vi "Install Dependencies.vi"(7 "Stored Install Data":path, 10 "Variant":variant) -> (0 "Error Out":errorcluster)   [LabVIEW 2011, in "LVH-Toolbox.lvlib" / "Installer Tools.lvlib"]
uses:
  Installer Tools.lvlib
  Private/Type Defs/Deps State.ctl
  <vilib>/Utility/file.llb/Read From Spreadsheet File (string).vi
  Private/Dependency Test VI Template.vi
  Common/LVH-Common.lvlib
panel:
  out "Tab Control":T1(tab)
  out "Package Name":string
  in  "Listbox":i32(listbox)
  in  "Info Cancel Button":bool
  in  "Info Next Button":bool
  out "Status":string
  out "Download Progress":u8(slide) scale=0.0..100.0
  in  "Multicolumn Listbox":i32(listbox)
  in  "Install Next":bool
  in  "Install Cancel":bool
  in  "Summary Finish":bool
  # "Testing Dependencies . . ."
  # "Select dependencies you want to install."
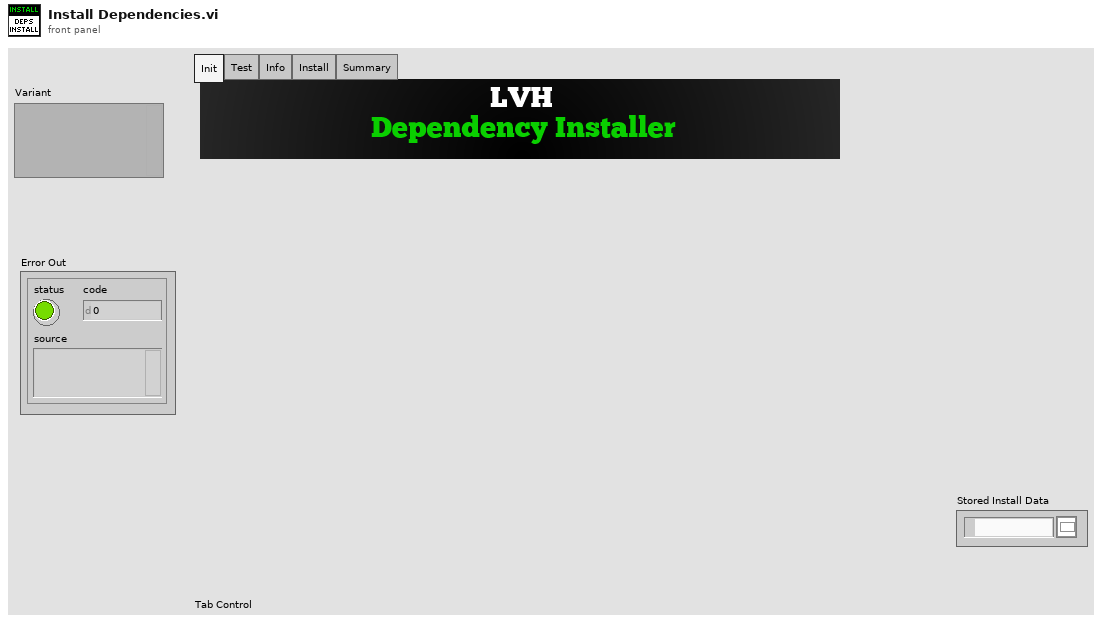
[diagram p1: front panel]
types:
  T1 = enum32{"Init", "Test", "Info", "Install", "Summary"}
  T2 = typedef "LVH-Toolbox.lvlib/Installer Tools.lvlib/Deps State.ctl" = enum16{"Init", "Test", "Info", "Install", "Summary"}
  T3 = typedef "LVH-Toolbox.lvlib/Installer Tools.lvlib/Dependency Config.ctl" = cluster{"Dependencies":T4[], "Files Installed":path[], "Dependency Config":path, "Installer Helper":path, "Dep Index":i32, "Download":T5}
  T4 = typedef "LVH-Toolbox.lvlib/Installer Tools.lvlib/Dependecy.ctl" = cluster{"Name":string, "Version":string, "Test VI Path":path, "Source URL":string, "Dep Met?":bool, "Install?":bool, "Installer Args":string}
  T5 = typedef "LVH-Toolbox.lvlib/LVH-Common.lvlib/Download Task.ctl" = cluster{"URL":string, "Local Path":path, "Download Worker":refnum<vi>, "Total Size (Bytes)":u64, "Prev Downloaded Size":u64, "Prev Download Time Stamp":timestamp}
  T6 = enum16{"Init", "Start DL", "Downloading", "DL Complete", "Done"}
  T7 = typedef "LVPoint32TypeDef.ctl" = cluster{"Horizontal":i32, "Vertical":i32}
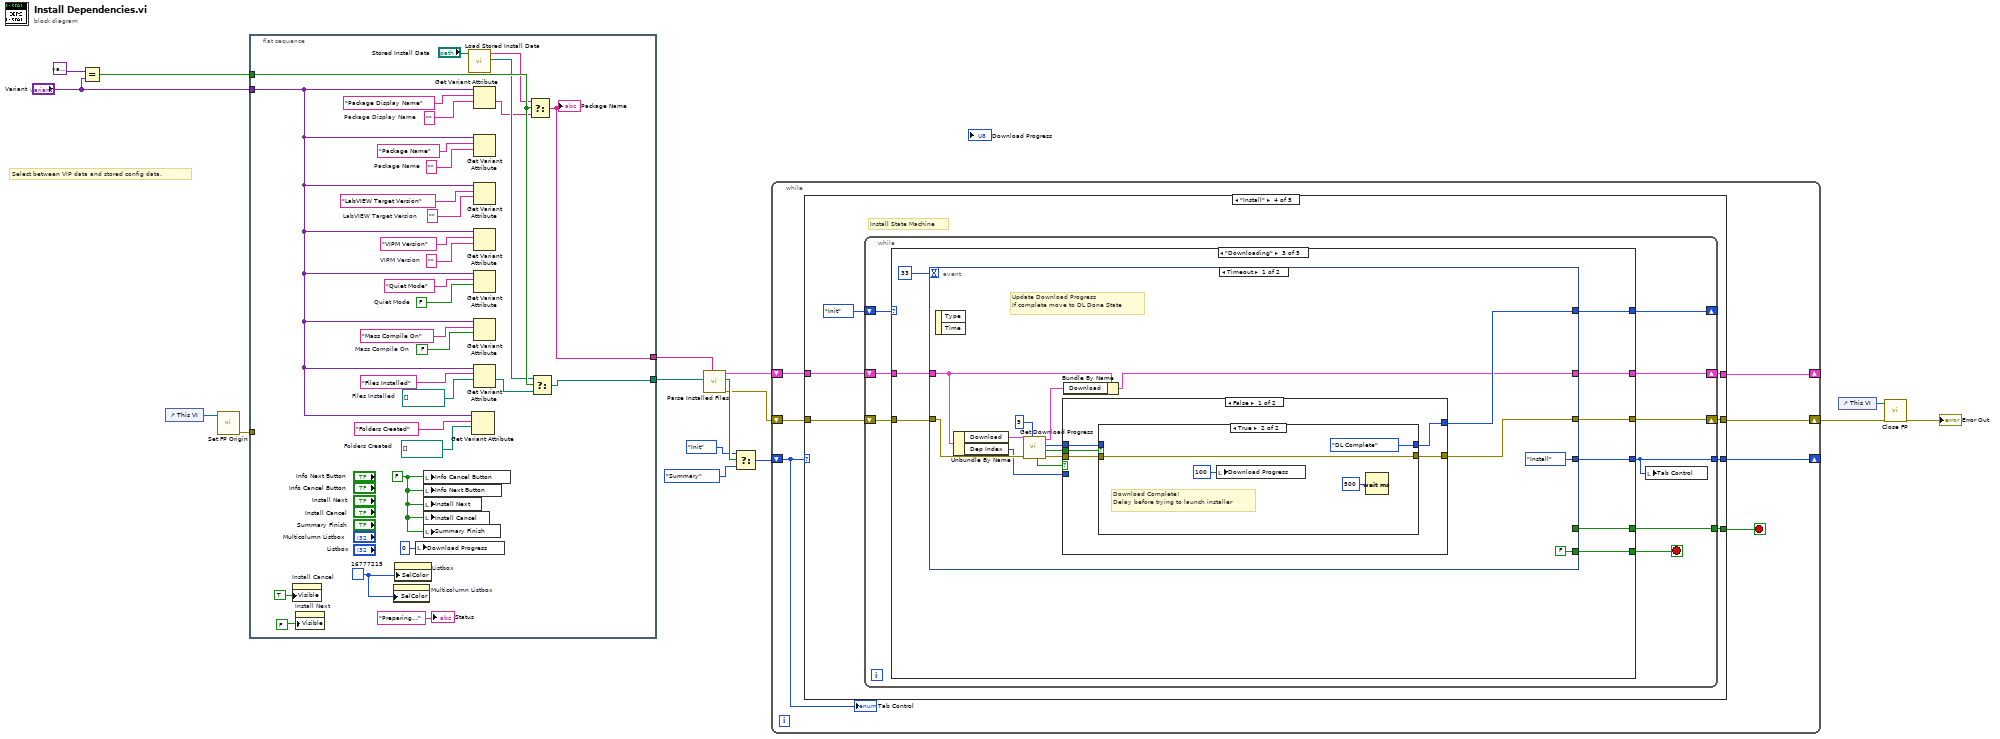
[diagram p0: block diagram]
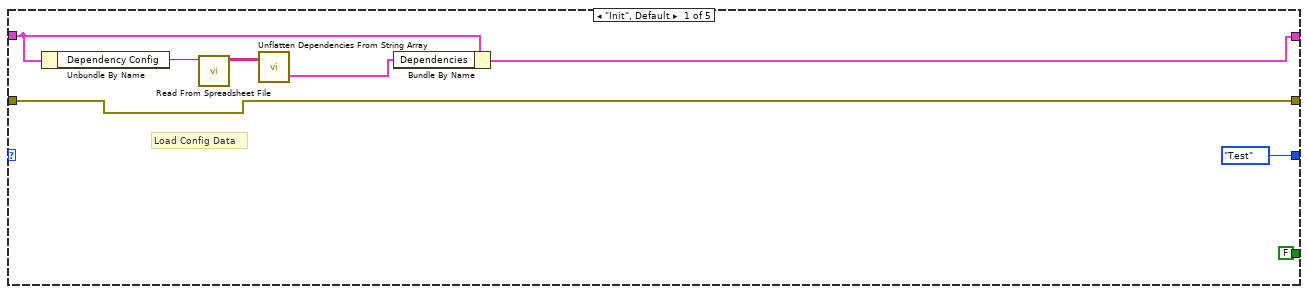
[diagram p2: hidden frame]
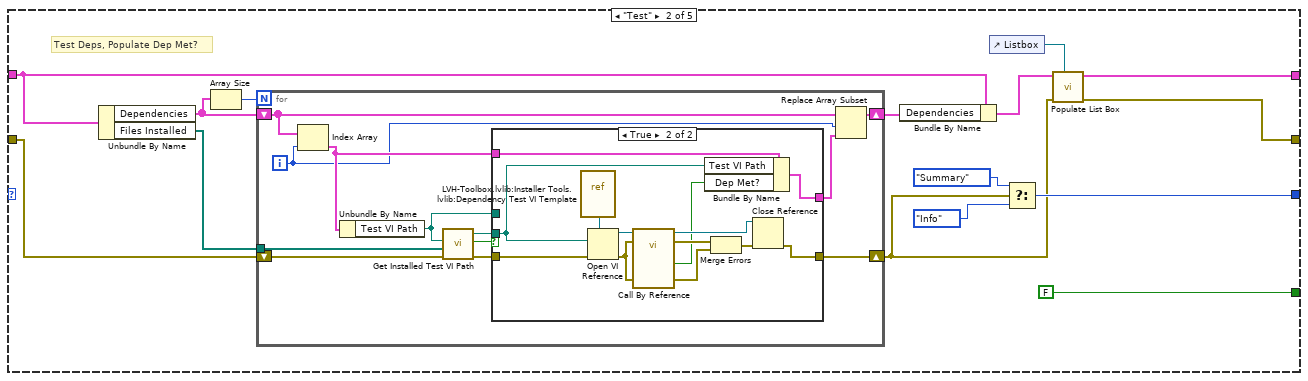
[diagram p3: hidden frame]
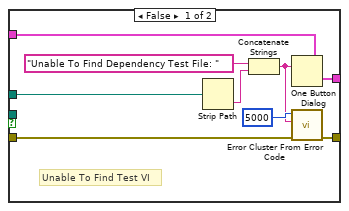
[diagram p4: hidden frame]
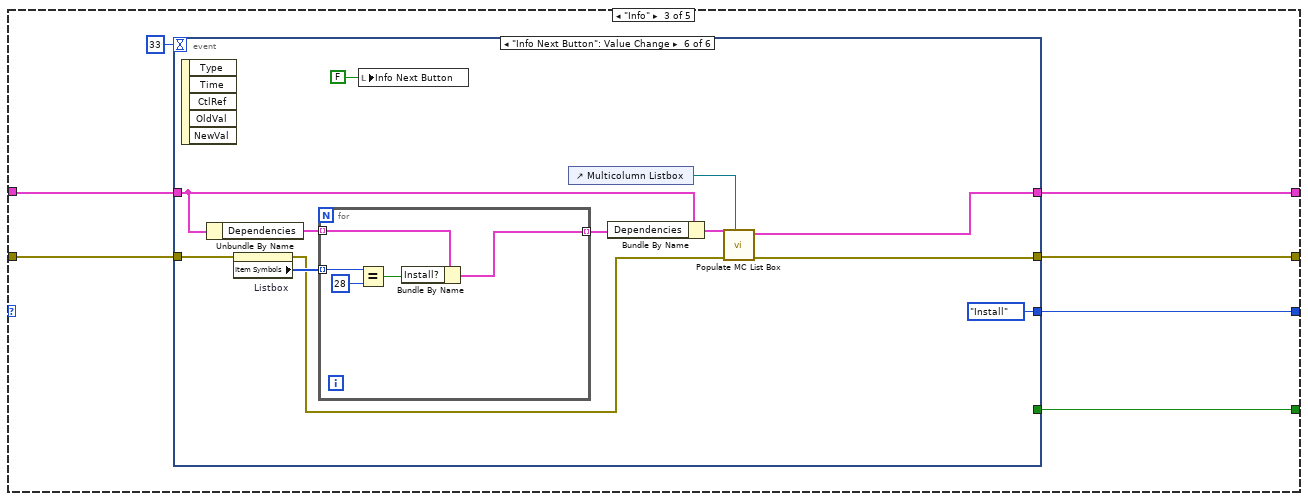
[diagram p5: hidden frame]
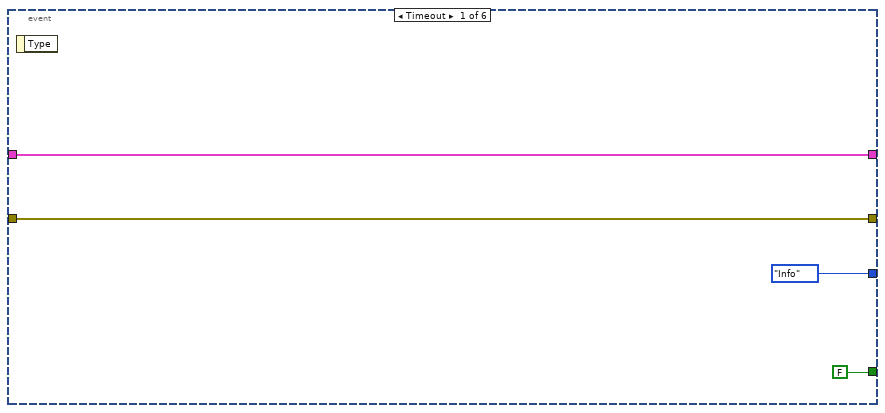
[diagram p6: hidden frame]
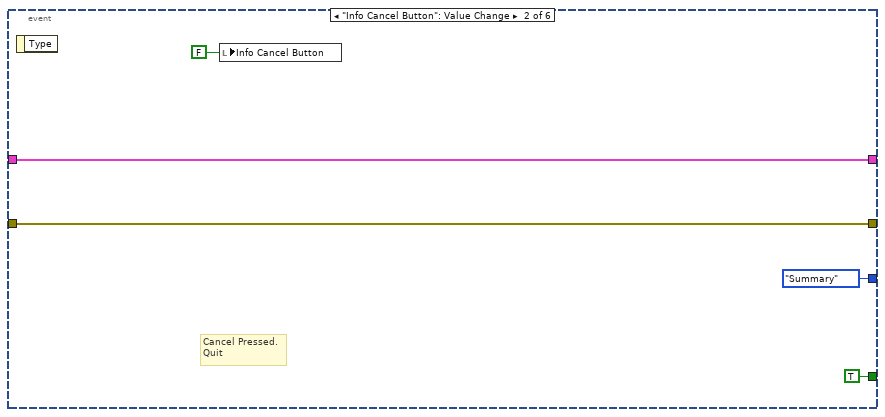
[diagram p7: hidden frame]
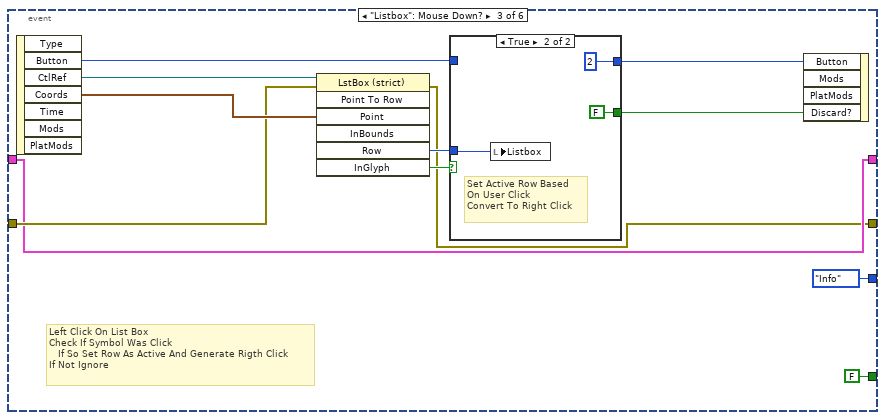
[diagram p8: hidden frame]
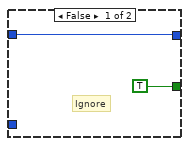
[diagram p9: hidden frame]
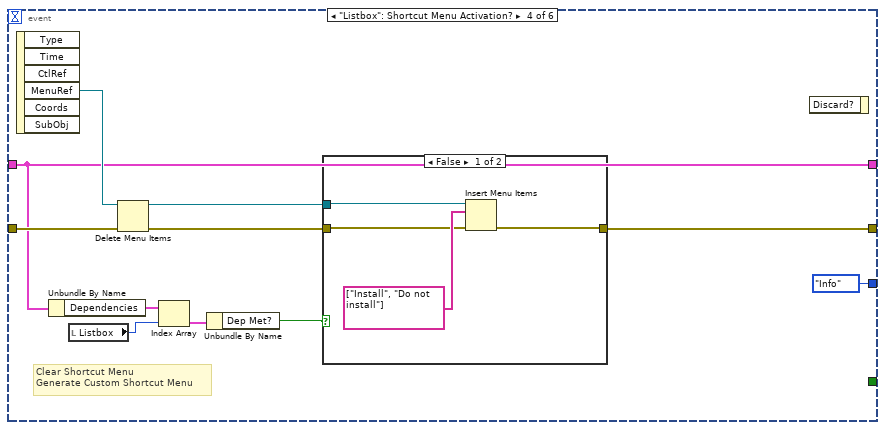
[diagram p10: hidden frame]
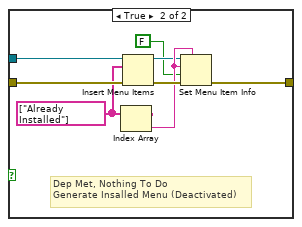
[diagram p11: hidden frame]
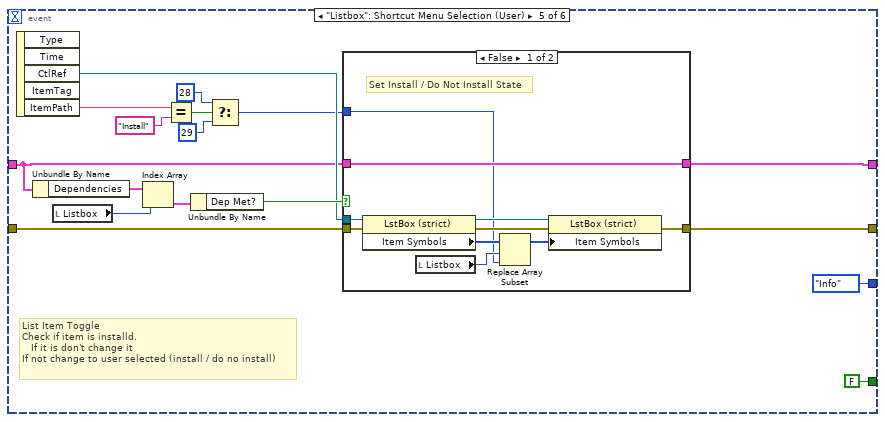
[diagram p12: hidden frame]
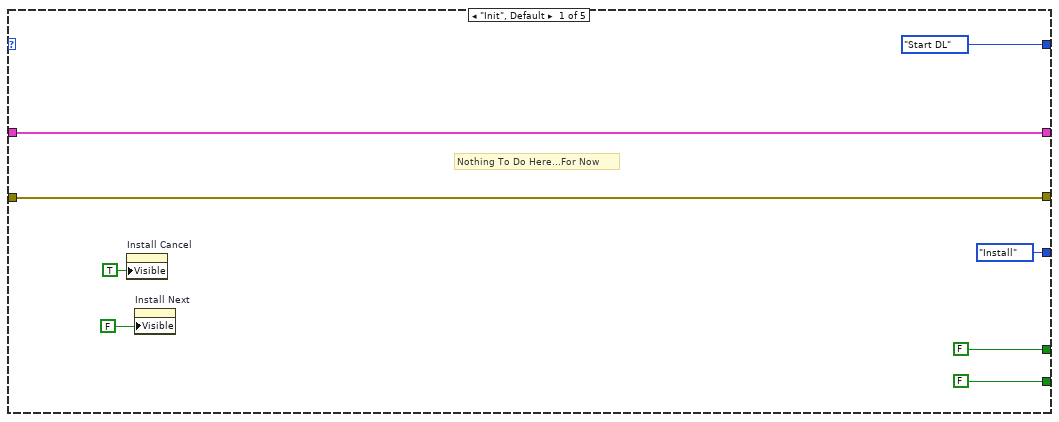
[diagram p14: hidden frame]
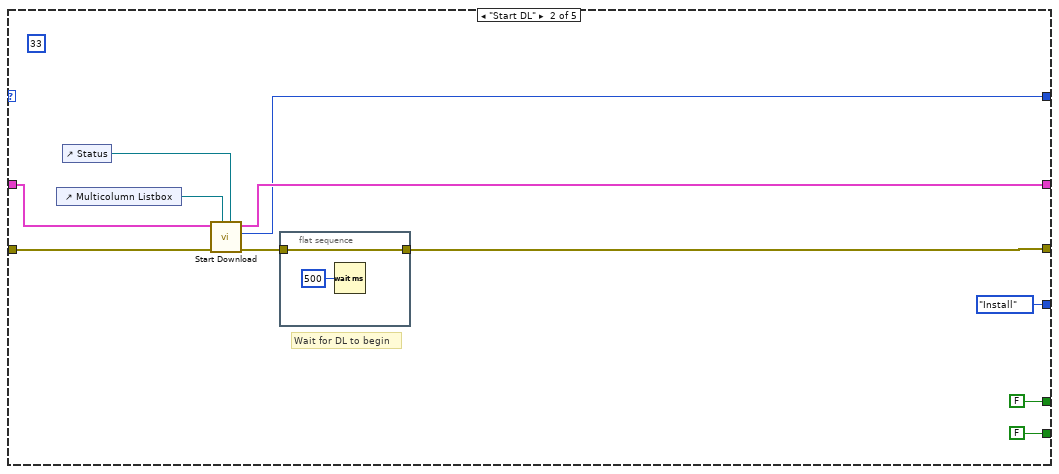
[diagram p15: hidden frame]
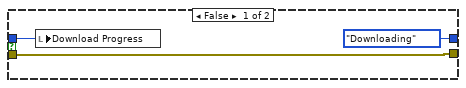
[diagram p16: hidden frame]
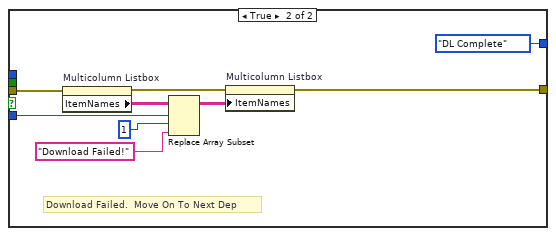
[diagram p17: hidden frame]
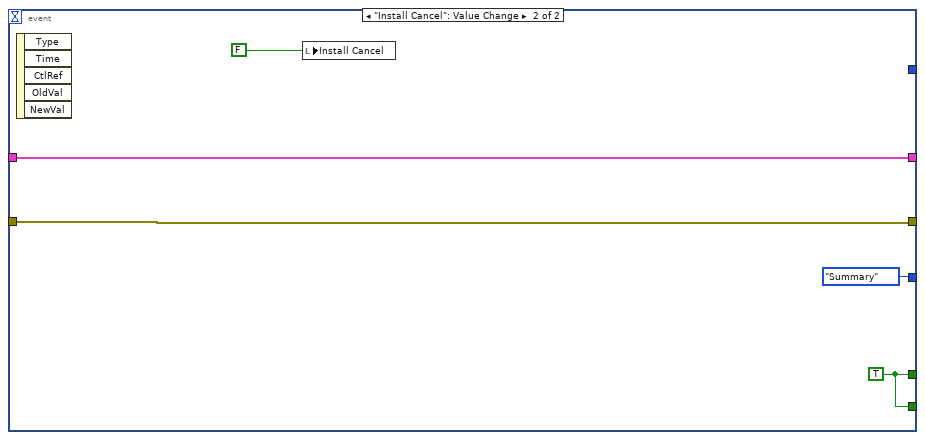
[diagram p18: hidden frame]
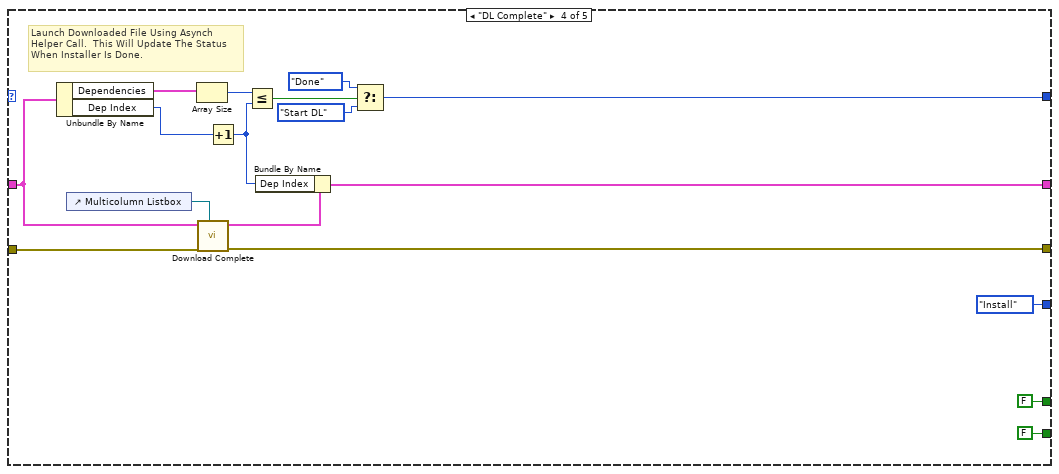
[diagram p19: hidden frame]
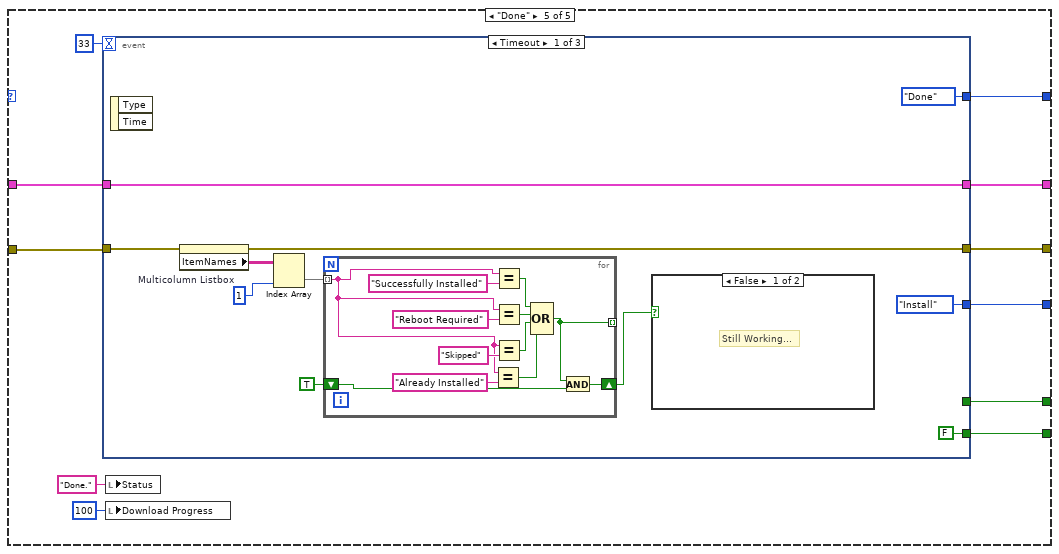
[diagram p20: hidden frame]
diagram:
  # "Select between VIP data and stored config data."
  n1 = Equal?(x=variant ("Variant"), y="Variant") -> (x = y?=w2:bool)
  n2 = control-ref of="This VI"() -> (w10:refnum<vi>)
  n3 = call "Set FP Origin.vi"("VI Ref"=w10) -> ("Error Out"=w11:errorcluster)  [unwired: 10 in]
  n4 = flat-sequence {
    tunnel: w11 -> [_]
    tunnel: "Variant" -> [w25]
    tunnel: [w21] -> w4
    tunnel: w2 -> [w24]
    tunnel: [w22] -> w1
    frame #0 {
      w31 = u32 16777215
      w29 = FALSE ("Cancel Button")
      w32 = path[] []  # Folders Created
      w33 = path[] []  # Files Installed
      w36 = FALSE  # Mass Compile On
      w37 = ""  # Package Display Name
      w38 = FALSE  # Quiet Mode
      w41 = ""  # VIPM Version
      w43 = ""  # LabVIEW Target Version
      w45 = ""  # Package Name
      n5 = property on="Install Cancel" class="Bool (strict)"("Visible"=TRUE) -> ()  [unwired: 2 in, 2 out]
      n6 = property on="Install Next" class="Bool (strict)"("Visible"=FALSE) -> ()  [unwired: 2 in, 2 out]
      n7 = property on="Multicolumn Listbox" class="MCListbox (strict)"("SelColor"=w31) -> ()  [unwired: 2 in, 2 out]
      n8 = property on="Listbox" class="LstBox (strict)"("SelColor"=w31) -> ()  [unwired: 2 in, 2 out]
      n9 = local write "Download Progress"(u8 0 ("Download Progress")) -> ()
      n10 = local write "Info Cancel Button"(w29) -> ()
      n11 = local write "Info Next Button"(w29) -> ()
      n12 = local write "Install Next"(w29) -> ()
      n13 = local write "Install Cancel"(w29) -> ()
      n14 = local write "Summary Finish"(w29) -> ()
      n15 = call "Load Stored Install Data.vi"("Stored Install Data"="Stored Install Data") -> ("Installed Files"=w20:path[], "Package Display Name"=w18:string)  [unwired: 9 in]
      n16 = Get Variant Attribute(Variant=w25, name="Folders Created", default value (empty Variant)=w32) -> ()  [unwired: 1 in, 4 out]
      n17 = Get Variant Attribute(Variant=w25, name="Package Display Name", default value (empty Variant)=w37) -> (value=w17:string)  [unwired: 1 in, 3 out]
      n18 = Get Variant Attribute(Variant=w25, name="Package Name", default value (empty Variant)=w45) -> ()  [unwired: 1 in, 4 out]
      n19 = Get Variant Attribute(Variant=w25, name="LabVIEW Target Version", default value (empty Variant)=w43) -> ()  [unwired: 1 in, 4 out]
      n20 = Get Variant Attribute(Variant=w25, name="VIPM Version", default value (empty Variant)=w41) -> ()  [unwired: 1 in, 4 out]
      n21 = Get Variant Attribute(Variant=w25, name="Quiet Mode", default value (empty Variant)=w38) -> ()  [unwired: 1 in, 4 out]
      n22 = Get Variant Attribute(Variant=w25, name="Mass Compile On", default value (empty Variant)=w36) -> ()  [unwired: 1 in, 4 out]
      n23 = Get Variant Attribute(Variant=w25, name="Files Installed", default value (empty Variant)=w33) -> (value=w19:path[])  [unwired: 1 in, 3 out]
      n24 = Select(t=w18, s=w24, f=w17) -> (s? t:f=w21:string)
      "Package Name" <- w21
      n25 = Select(t=w20, s=w24, f=w19) -> (s? t:f=w22:path[])
      "Status" <- "Preparing..." ("Status")
    }
  }
  n26 = call "Parse Installed Files.vi"("Package Name"=w4, "Files Installed"=w1) -> ("Error Out"=w9:errorcluster, "Config Found?"=w16:bool, "Dependecy Config out"=w12:T3)  [unwired: 7 in]
  n27 = Select(t=Deps_State."Init" ("Deps State"), s=w16, f=Deps_State."Summary" ("Deps State")) -> (s? t:f=w13:T2)
  n28 = while {
    shift-right: [w50] -> _
    shift-left: w13 -> [w48]
    shift-right: [w54] -> _
    shift-left: w12 -> [w53]
    shift-right: [w51] -> w7
    shift-left: w9 -> [w52]
    stop <- w49 stop-if-true
    n29 = case shown="\"Install\"" w48 {
      tunnel: [w61 w66 w112 w216 w368] -> w54
      tunnel: w53 -> [w60 w73 w117 w219 w367]
      tunnel: w52 -> [w58 w76 w115 w218 w370]
      tunnel: [w58 w63 w116 w217 w369] -> w51
      tunnel: [Deps_State."Test" ("Deps State") w69 w114 w213 Deps_State."Summary" ("Deps State")] -> w50
      tunnel: [FALSE FALSE w113 w214 w371] -> w49
      frame "Init", Default {
        # "Load Config Data"
        n30 = Unbundle By Name(w60) -> ("Dependency Config"=w59:path)
        n31 = call-poly <vilib>:"Read From Spreadsheet File.vi"("file path (dialog if empty)"=w59) -> ("all rows"=w62:string[][])  [unwired: 6 in, 4 out]
        n32 = call "Unflatten Dependencies From String Array.vi"("Flattened Dependencies"=w62) -> ("Deps"=w55:T4[])  [unwired: 1 in, 1 out]
        n33 = Bundle By Name(cluster=w60, "Dependencies"=w55) -> (w61:T3)
      }
      frame "Test" {
        # "Test Deps, Populate Dep Met?"
        n34 = Unbundle By Name(w73) -> ("Dependencies"=w74:T4[], "Files Installed"=w77:path[])
        n35 = Array Size(array=w74) -> (size(s)=w75:i32)
        n36 = for {
          N: w75 -> [_]
          tunnel: w77 -> [w89]
          shift-right: [w80] -> w65
          shift-left: w76 -> [w88]
          shift-right: [w83] -> w72
          shift-left: w74 -> [w82]
          i -> [w79]
          n37 = Index Array(array=w82, index=w79) -> (element=w84:T4)
          n38 = Unbundle By Name(w84) -> ("Test VI Path"=w78:path)
          n39 = call "Get Installed Test VI Path.vi"("Error In"=w88, "Files Installed"=w89, "Test VI Path"=w78) -> ("Error Out"=w87:errorcluster, "Found?"=w85:bool, "Installed Test VI Path"=w86:path)  [unwired: 6 in]
          n40 = case shown="True" w85 {
            tunnel: w87 -> [w95 w110]
            tunnel: w86 -> [_ w98]
            tunnel: [w97 w101] -> w81
            tunnel: w84 -> [w97 w100]
            tunnel: [w94 w99] -> w80
            tunnel: w78 -> [w90 _]
            frame False {
              # "Unable To Find Test VI"
              n41 = Strip Path(path=w90) -> (name=w92:string)  [unwired: 1 out]
              n42 = Concatenate Strings("Unable To Find Dependency Test File: " ("message"), w92) -> (w91:string)
              n43 = One Button Dialog(message=w91) -> ()  [unwired: 1 in, 1 out]
              n44 = call <vilib>:"Error Cluster From Error Code.vi"("error in (no error)"=w95, "error message (\"\")"=w91, "error code (0)"=5000) -> ("error out"=w94:errorcluster)  [unwired: 6 in]
            }
            frame True {
              n45 = vi-ref "LVH-Toolbox.lvlib:Installer Tools.lvlib:Dependency Test VI Template.vi"() -> (w108:refnum<vi>)
              n46 = Open VI Reference(type specifier VI Refnum (for type only)=w108, vi path=w98, error in (no error)=w110) -> (vi reference=w109:refnum<vi>, error out=w107:errorcluster)  [unwired: 3 in]
              n47 = call-by-ref "?"(reference=w109, error in=w107, "Error In"=w107) -> (reference out=w103:refnum<vi>, error out=w106:errorcluster, "Error Out"=w105:errorcluster, "Pass?"=w102:bool)  [unwired: 9 in]
              n48 = Bundle By Name(cluster=w100, "Test VI Path"=w98, "Dep Met?"=w102) -> (w101:T4)
              n49 = Merge Errors(w106, w105) -> (w104:errorcluster)
              n50 = Close Reference(reference=w103, error in (no error)=w104) -> (error out=w99:errorcluster)
            }
          }
          n51 = Replace Array Subset(array=w82, new element=w81, index=w79) -> (w83:T4[])
        }
        n52 = Bundle By Name(cluster=w73, "Dependencies"=w72) -> (w67:T3)
        n53 = control-ref of="Listbox"() -> (w64:refnum<vi>)
        n54 = Select(t=Deps_State."Summary" ("Deps State"), s=w65, f=Deps_State."Info" ("Deps State")) -> (s? t:f=w69:T2)
        n55 = call "Populate List Box.vi"("Listbox Ref"=w64, "Error In"=w65, "Dependecy Config"=w67) -> ("Error Out"=w63:errorcluster, "Dependecy Config"=w66:T3)  [unwired: 7 in]
      }
      frame "Info" {
        n56 = event shown="[5] \"Info Next Button\": Value Change" {
          selector: _ -> [_ _ _ _ _ _]
          dyn-events: _ -> [_ _ _ _ _ _]
          timeout: 33 -> [_ _ _ _ _ _]
          tunnel: w117 -> [w118 w122 w130 w146 w168 w200]
          tunnel: [w119 w123 w128 w145 w170 w196] -> w116
          tunnel: w115 -> [w119 w123 w136 w154 w175 w201]
          tunnel: [Deps_State."Info" ("Deps State") Deps_State."Summary" ("Deps State") Deps_State."Info" ("Deps State") Deps_State."Info" ("Deps State") Deps_State."Info" ("Deps State") Deps_State."Install" ("Deps State")] -> w114
          tunnel: [FALSE TRUE FALSE _ FALSE _] -> w113
          tunnel: [w118 w122 w130 w146 w169 w205] -> w112
          event Timeout {
            n57 = event-data() -> ()  [unwired: 1 in, 1 out]
          }
          event "Info Cancel Button": Value Change {
            # "Cancel Pressed.\nQuit"
            n58 = event-data() -> ()  [unwired: 1 in, 1 out]
            n59 = local write "Info Cancel Button"(FALSE ("Cancel Button")) -> ()
          }
          event "Listbox": Mouse Down? {
            # "Left Click On List Box\nCheck If Symbol Was Click\n   If So Set Row As Active And Generate Rigth Click\nIf Not Ignore"
            n60 = event-data() -> ("Button"=w131:u16, "CtlRef"=w138:refnum<vi>, "Coords"=w137:T7)  [unwired: 1 in, 4 out]
            n61 = invoke class="LstBox (strict)" method="Point To Row"(reference=w138, error in=w136, "Point"=w137) -> (error out=w128:errorcluster, "Row"=w133:i32, "InGlyph"=w135:bool)  [unwired: 4 in, 4 out]
            n62 = case shown="True" w135 {
              tunnel: w133 -> [_ w142]
              tunnel: [w140 u16 2 ("Button")] -> w132
              tunnel: w131 -> [w140 _]
              tunnel: [TRUE FALSE] -> w127
              frame False {
                # "Ignore"
              }
              frame True {
                # "Set Active Row Based \nOn User Click\nConvert To Right Click"
                n63 = local write "Listbox"(w142) -> ()
              }
            }
            n64 = event-data("Button"=w132, "Discard?"=w127) -> ()  [unwired: 3 in, 1 out]
          }
          event "Listbox": Shortcut Menu Activation? {
            # "Clear Shortcut Menu\nGenerate Custom Shortcut Menu"
            n65 = event-data() -> ("MenuRef"=w153:refnum<k9>)  [unwired: 1 in, 5 out]
            n66 = Unbundle By Name(w146) -> ("Dependencies"=w149:T4[])
            n67 = local read "Listbox"() -> (w148:i32)
            n68 = Delete Menu Items(6:w154, 9:w153) -> (0:w151:errorcluster, 3:w150:refnum<k9>)  [unwired: 2 in]
            n69 = Index Array(array=w149, index=w148) -> (element=w147:T4)
            n70 = Unbundle By Name(w147) -> ("Dep Met?"=w144:bool)
            n71 = case shown="False" w144 {
              tunnel: w151 -> [w157 w166]
              tunnel: w150 -> [w156 w165]
              tunnel: [w155 w163] -> w145
              frame False {
                n72 = Insert Menu Items(6:w157, 8:string[] ["Install", "Do not install"], 9:w156) -> (0:w155:errorcluster)  [unwired: 3 in, 2 out]
              }
              frame True {
                w162 = string[] ["Already Installed"] ("item names")
                # "Dep Met, Nothing To Do\nGenerate Insalled Menu (Deactivated)"
                n73 = Index Array(array=w162) -> (element=w161:string)  [unwired: 1 in]
                n74 = Insert Menu Items(6:w166, 8:w162, 9:w165) -> (0:w164:errorcluster, 3:w160:refnum<k9>)  [unwired: 3 in, 1 out]
                n75 = Set Menu Item Info(7:w161, 8:w164, 9:FALSE ("enabled"), 10:w161, 11:w160) -> (0:w163:errorcluster)  [unwired: 2 in, 1 out]
              }
            }
            n76 = event-data() -> ()  [unwired: 2 in, 1 out]
          }
          event "Listbox": Shortcut Menu Selection (User) {
            # "List Item Toggle\nCheck if item is installd.\n   If it is don't change it\nIf not change to user selected (install / do no install)"
            n77 = event-data() -> ("CtlRef"=w176:refnum<vi>, "ItemPath"=w182:string)  [unwired: 1 in, 3 out]
            n78 = Unbundle By Name(w168) -> ("Dependencies"=w180:T4[])
            n79 = local read "Listbox"() -> (w179:i32)
            n80 = Index Array(array=w180, index=w179) -> (element=w178:T4)
            n81 = Equal?(x=w182, y="Install") -> (x = y?=w174:bool)
            n82 = Unbundle By Name(w178) -> ("Dep Met?"=w177:bool)
            n83 = Select(t=28, s=w174, f=29 ("t")) -> (s? t:f=w171:i32)
            n84 = case shown="False" w177 {
              tunnel: w176 -> [w193 _]
              tunnel: w175 -> [w192 w195]
              tunnel: w171 -> [w184 _]
              tunnel: [w187 w195] -> w170
              tunnel: [w186 w194] -> w169
              tunnel: w168 -> [w186 w194]
              frame False {
                # "Set Install / Do Not Install State"
                n85 = property class="LstBox (strict)"(reference=w193, error in=w192) -> (reference out=w191:refnum<vi>, error out=w190:errorcluster, "Item Symbols"=w189:i32[])
                n86 = local read "Listbox"() -> (w185:i32)
                n87 = Replace Array Subset(array=w189, new element=w184, index=w185) -> (w188:i32[])
                n88 = property class="LstBox (strict)"(reference=w191, error in=w190, "Item Symbols"=w188) -> (error out=w187:errorcluster)  [unwired: 1 out]
              }
              frame True {
                # "Dependency is installd.   Leave it alone."
              }
            }
          }
          event "Info Next Button": Value Change {
            n89 = event-data() -> ()  [unwired: 1 in, 5 out]
            n90 = Unbundle By Name(w200) -> ("Dependencies"=w203:T4[])
            n91 = property on="Listbox" class="LstBox (strict)"(error in=w201) -> (error out=w197:errorcluster, "Item Symbols"=w202:i32[])  [unwired: 1 in, 1 out]
            n92 = for {
              tunnel: w203 -> [w209] mode=indexing
              tunnel: w202 -> [w211] mode=indexing
              tunnel: [w208] -> w199 mode=indexing
              n93 = Equal?(x=w211, y=28) -> (x = y?=w210:bool)
              n94 = Bundle By Name(cluster=w209, "Install?"=w210) -> (w208:T4)
            }
            n95 = local write "Info Next Button"(FALSE ("Next Button")) -> ()
            n96 = control-ref of="Multicolumn Listbox"() -> (w204:refnum<vi>)
            n97 = Bundle By Name(cluster=w200, "Dependencies"=w199) -> (w198:T3)
            n98 = call "Populate MC List Box.vi"("Listbox Ref"=w204, "Error In"=w197, "Dependecy Config"=w198) -> ("Error Out"=w196:errorcluster, "Dependecy Config"=w205:T3)  [unwired: 7 in]
          }
        }
      }
      frame "Install" {
        # "Install State Machine"
        n99 = while {
          shift-right: [w221] -> _
          shift-left: T6."Init" ("Install State") -> [w223]
          tunnel: [w222] -> w214
          tunnel: [w220] -> w213
          shift-right: [w225] -> w216
          shift-left: w219 -> [w228]
          shift-right: [w226] -> w217
          shift-left: w218 -> [w227]
          stop <- w224 stop-if-true
          n100 = case shown="\"Downloading\"" w223 {
            tunnel: w228 -> [w233 w242 w258 w307 w327]
            tunnel: w227 -> [w234 w247 w257 w313 w320]
            tunnel: [w234 w238 w256 w314 w326] -> w226
            tunnel: [w233 w241 w255 w303 w325] -> w225
            tunnel: [FALSE FALSE w253 FALSE w323] -> w224
            tunnel: [FALSE FALSE w252 FALSE w322] -> w222
            tunnel: [Deps_State."Install" ("Deps State") Deps_State."Install" ("Deps State") w251 Deps_State."Install" ("Deps State") w321] -> w220
            tunnel: [T6."Start DL" ("Install State") w240 w250 w302 w317] -> w221
            frame "Init", Default {
              # "Nothing To Do Here...For Now"
              n101 = property on="Install Cancel" class="Bool (strict)"("Visible"=TRUE) -> ()  [unwired: 2 in, 2 out]
              n102 = property on="Install Next" class="Bool (strict)"("Visible"=FALSE) -> ()  [unwired: 2 in, 2 out]
            }
            frame "Start DL" {
              (unwired) 33
              # "Wait for DL to begin"
              n103 = control-ref of="Multicolumn Listbox"() -> (w243:refnum<vi>)
              n104 = control-ref of="Status"() -> (w244:refnum<vi>)
              n105 = call "Start Download.vi"("Overall Status"=w244, "Itemized Status"=w243, "Error In"=w247, "Dependecy Config"=w242) -> ("Error Out"=w237:errorcluster, "Install State"=w240:T6, "Dependecy Config"=w241:T3)  [unwired: 5 in]
              n106 = flat-sequence {
                tunnel: [w248] -> w238
                tunnel: w237 -> [w248]
                frame #0 {
                  n107 = Wait (ms)(milliseconds to wait=u32 500) -> ()  [unwired: 1 out]
                }
              }
            }
            frame "Downloading" {
              n108 = event shown="[0] Timeout" {
                selector: _ -> [_ _]
                dyn-events: _ -> [_ _]
                timeout: 33 -> [_ _]
                tunnel: w258 -> [w262 w296]
                tunnel: [w268 w295] -> w256
                tunnel: w257 -> [w272 w295]
                tunnel: [FALSE w298] -> w253
                tunnel: [w261 w296] -> w255
                tunnel: [_ w298] -> w252
                tunnel: [Deps_State."Install" ("Deps State") Deps_State."Summary" ("Deps State")] -> w251
                tunnel: [w266 _] -> w250
                event Timeout {
                  # "Update Download Progress\nIf complete move to DL Done State"
                  n109 = event-data() -> ()  [unwired: 1 in, 2 out]
                  n110 = Unbundle By Name(w262) -> ("Download"=w264:T5, "Dep Index"=w260:i32)
                  n111 = call "Get Download Progress.vi"("Download Timeout (S)"=u32 5, "Error In"=w272, "Download"=w264) -> ("Error Out"=w269:errorcluster, "Complete?"=w267:bool, "Percent Complete"=w265:i32, "Download"=w263:T5, "Timeout?"=w270:bool)  [unwired: 4 in]
                  n112 = case shown="False" w270 {
                    tunnel: w269 -> [w276 w294]
                    tunnel: [w275 w289] -> w268
                    tunnel: w267 -> [w278 _]
                    tunnel: [w277 T6."DL Complete" ("Install State")] -> w266
                    tunnel: w265 -> [w274 _]
                    tunnel: w260 -> [_ w286]
                    frame False {
                      n113 = case shown="True" w278 {
                        tunnel: [T6."Downloading" ("Install State") T6."DL Complete" ("Install State")] -> w277
                        tunnel: w276 -> [w280 w283]
                        tunnel: [w280 w283] -> w275
                        tunnel: w274 -> [w281 _]
                        frame False {
                          n114 = local write "Download Progress"(w281) -> ()
                        }
                        frame True {
                          # "Download Complete!\nDelay before trying to launch installer"
                          n115 = local write "Download Progress"(u8 100 ("Download Progress")) -> ()
                          n116 = Wait (ms)(milliseconds to wait=u32 500) -> ()  [unwired: 1 out]
                        }
                      }
                    }
                    frame True {
                      # "Download Failed.  Move On To Next Dep"
                      n117 = property on="Multicolumn Listbox" class="MCListbox (strict)"(error in=w294) -> (error out=w291:errorcluster, "ItemNames"=w293:string[][])  [unwired: 1 in, 1 out]
                      n118 = Replace Array Subset(array=w293, new element="Download Failed!" ("new element/subarray"), index (row)=w286, index (col)=1 ("disabled index (col)")) -> (w290:string[][])
                      n119 = property on="Multicolumn Listbox" class="MCListbox (strict)"(error in=w291, "ItemNames"=w290) -> (error out=w289:errorcluster)  [unwired: 1 in, 1 out]
                    }
                  }
                  n120 = Bundle By Name(cluster=w262, "Download"=w263) -> (w261:T3)
                }
                event "Install Cancel": Value Change {
                  w298 = TRUE
                  n121 = event-data() -> ()  [unwired: 1 in, 5 out]
                  n122 = local write "Install Cancel"(FALSE ("Cancel Button")) -> ()
                }
              }
            }
            frame "DL Complete" {
              # "Launch Downloaded File Using Asynch\nHelper Call.  This Will Update The Status\nWhen Installer Is Done."
              n123 = Unbundle By Name(w307) -> ("Dependencies"=w306:T4[], "Dep Index"=w305:i32)
              n124 = control-ref of="Multicolumn Listbox"() -> (w312:refnum<vi>)
              n125 = Array Size(array=w306) -> (size(s)=w308:i32)
              n126 = call "Download Complete.vi"("MulticolumnListbox in"=w312, "Error In"=w313, "Dependency Config"=w307) -> ("Error Out"=w314:errorcluster, "Dependency Config"=w304:T3)  [unwired: 7 in]
              n127 = Increment(x=w305) -> (x+1=w301:i32)
              n128 = Less Or Equal?(x=w308, y=w301) -> (x <= y?=w311:bool)
              n129 = Bundle By Name(cluster=w304, "Dep Index"=w301) -> (w303:T3)
              n130 = Select(t=T6."Done" ("Install State"), s=w311, f=T6."Start DL" ("Install State")) -> (s? t:f=w302:T6)
            }
            frame "Done" {
              n131 = event shown="[0] Timeout" {
                selector: _ -> [_ _ _]
                dyn-events: _ -> [_ _ _]
                timeout: 33 -> [_ _ _]
                tunnel: w327 -> [w334 w356 w363]
                tunnel: [w333 w358 w364] -> w326
                tunnel: w320 -> [w335 w358 w364]
                tunnel: [FALSE TRUE w362] -> w323
                tunnel: [w334 w356 w363] -> w325
                tunnel: [_ TRUE w362] -> w322
                tunnel: [Deps_State."Install" ("Deps State") Deps_State."Summary" ("Deps State") Deps_State."Summary" ("Deps State")] -> w321
                tunnel: [T6."Done" ("Install State") T6."Done" ("Install State") T6."Done" ("Install State")] -> w317
                event Timeout {
                  n132 = event-data() -> ()  [unwired: 1 in, 2 out]
                  n133 = property on="Multicolumn Listbox" class="MCListbox (strict)"(error in=w335) -> (error out=w333:errorcluster, "ItemNames"=w332:string[][])  [unwired: 1 in, 1 out]
                  n134 = Index Array(array=w332, index (col)=1 ("index (row)")) -> (element=w331:string[])  [unwired: 1 in]
                  n135 = for {
                    tunnel: w331 -> [w340] mode=indexing
                    tunnel: [w346] -> _ mode=indexing
                    shift-right: [w345] -> w329
                    shift-left: TRUE -> [w344]
                    n136 = Equal?(x=w340, y="Already Installed") -> (x = y?=w339:bool)
                    n137 = Equal?(x=w340, y="Successfully Installed") -> (x = y?=w348:bool)
                    n138 = Equal?(x=w340, y="Reboot Required") -> (x = y?=w347:bool)
                    n139 = Equal?(x=w340, y="Skipped") -> (x = y?=w342:bool)
                    n140 = Compound Arithmetic op=OR(w348, w347, w342, w339) -> (w346:bool)
                    n141 = And(x=w346, y=w344) -> (x .and. y?=w345:bool)
                  }
                  n142 = case shown="False" w329 {
                    frame False {
                      # "Still Working..."
                    }
                    frame True {
                      # "Done"
                      n143 = property on="Install Cancel" class="Bool (strict)"("Visible"=FALSE) -> ()  [unwired: 2 in, 2 out]
                      n144 = property on="Install Next" class="Bool (strict)"("Visible"=TRUE) -> ()  [unwired: 2 in, 2 out]
                    }
                  }
                }
                event "Install Next": Value Change {
                  n145 = event-data() -> ()  [unwired: 1 in, 5 out]
                  n146 = local write "Install Next"(FALSE ("Next Button")) -> ()
                }
                event "Install Cancel": Value Change {
                  w362 = TRUE
                  n147 = event-data() -> ()  [unwired: 1 in, 5 out]
                  n148 = local write "Install Cancel"(FALSE ("Cancel Button")) -> ()
                }
              }
              n149 = local write "Status"("Done." ("Status")) -> ()
              n150 = local write "Download Progress"(u8 100 ("Download Progress")) -> ()
            }
          }
          n151 = local write "Tab Control"(w220) -> ()
        }
      }
      frame "Summary" {
        n152 = event shown="[1] \"Summary Finish\": Value Change" {
          selector: _ -> [_ _]
          dyn-events: _ -> [_ _]
          timeout: 33 -> [_ _]
          tunnel: [FALSE TRUE] -> w371
          tunnel: w370 -> [w374 w377]
          tunnel: [w374 w377] -> w369
          tunnel: [w373 w376] -> w368
          tunnel: w367 -> [w373 w376]
          event Timeout {
            n153 = event-data() -> ()  [unwired: 1 in, 2 out]
          }
          event "Summary Finish": Value Change {
            n154 = event-data() -> ()  [unwired: 1 in, 5 out]
            n155 = local write "Summary Finish"(FALSE ("Cancel Button")) -> ()
          }
        }
      }
    }
    "Tab Control" <- w48
  }
  n156 = control-ref of="This VI"() -> (w8:refnum<vi>)
  n157 = call "Close FP.vi"("Error In"=w7, "VI Ref"=w8) -> ("Error Out"=→"Error Out":errorcluster)  [unwired: 9 in]
